vi "RSZVB Set Frequency Stimulus.vi"(8 "error in (no error)":errorcluster {"code" format="%.0x"}, 9 "Frequency Stimulus":string, 10 "Channel (1)":i32=1, 11 "VISA session":refnum<visa-resource-name>) -> (0 "error out":errorcluster {"code" format="%.0x"}, 3 "dup VISA session":refnum<visa-resource-name>)   [LabVIEW 2011]
doc: "This VI selects the stimulus signal that is used for the definition of the frequency sweep range or CW frequency. \n\nNote(s):\n\n(1) This command is particularly useful in arbitrary mode (with option R&S ZVA-K4), where the frequencies and source powers at the ports are independent. \n\n(2) For R&S ZVA and ZVT analyzers without option R&S ZVA-K4, all powers are coupled so that this selection has no effect. \n\n(3) For R&S ZVB analyzers, all frequencies are coupled so that this selection has no effect. \n\nRemote-control command(s):\n[SENSe<Ch>:]SWEep:AXIS:FREQuency '<frequency_ref>'"
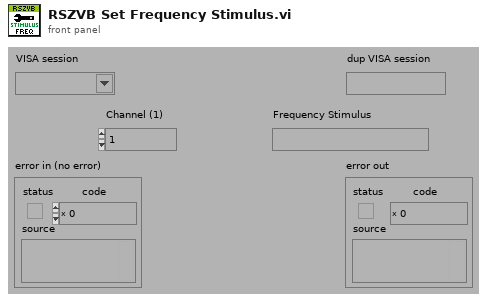
[diagram p1: front panel]
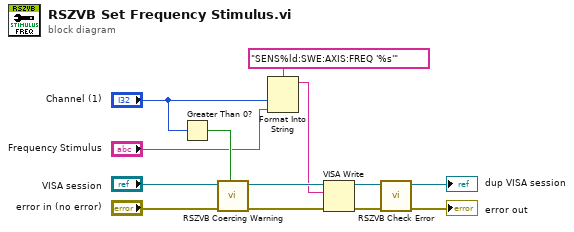
[diagram p0: block diagram]
diagram:
  n1 = Greater Than 0?(x="Channel (1)") -> (x > 0?=w7:bool)
  n2 = call "RSZVB Coercing Warning.vi"("In Range?"=w7, "error in (no error)"="error in (no error)", "VISA session"="VISA session") -> ("error out"=w11:errorcluster, "dup VISA session"=w12:refnum<visa-resource-name>)  [unwired: 7 in]
  n3 = Format Into String(format string="SENS%ld:SWE:AXIS:FREQ '%s'", "Channel (1)", "Frequency Stimulus") -> (resulting string=w8:string)  [unwired: 2 in, 1 out]
  n4 = VISA Write(VISA resource name=w12, write buffer=w8, error in (no error)=w11) -> (VISA resource name out=w9:refnum<visa-resource-name>, error out=w10:errorcluster)  [unwired: 1 out]
  n5 = call "RSZVB Check Error.vi"("error in (no error)"=w10, "VISA session"=w9) -> ("error out"=→"error out":errorcluster, "dup VISA session"=→"dup VISA session":refnum<visa-resource-name>)  [unwired: 8 in]
